vi "Control Panel Controller.vi"(8 "error in":errorcluster) -> ()   [LabVIEW 2020]
doc: "This VI executes continuously carrying out the current operation and responding to updates or new operations. It will often contain the timing or control code that is difficult to place directly in TeleOp. This VI generally opens all sensors and motors and isolates the rest of the robot code from knowing how the operations are carried out."
uses:
  Control Panel Operations.ctl
  Control Panel Setpoints.ctl
  <vilib>/Rock Robotics/Network Tables/NT Write Boolean.vi
  <vilib>/Rock Robotics/WPI/Framework/Completion Status.ctl
panel:
  in  "Interactive Values":T1
  out "Current\nCmd":string
  in  "Buttons":cluster{"Execute Cmd":bool, "Abort Cmd":bool}
  out "Command Timing":cluster{"Start Time (ms)":u32, "Iterations":i32}
  out "Status":T3
  # "Tip: It may be helpful to observe inputs and sensor values.\nYou may also want to display tuning or debugging controls."
  # "Interactive Command: You may fill in the settings for a command\nand schedule it with the Execute button. You can observe and abort\nany command while fine tuning the code for the controller."
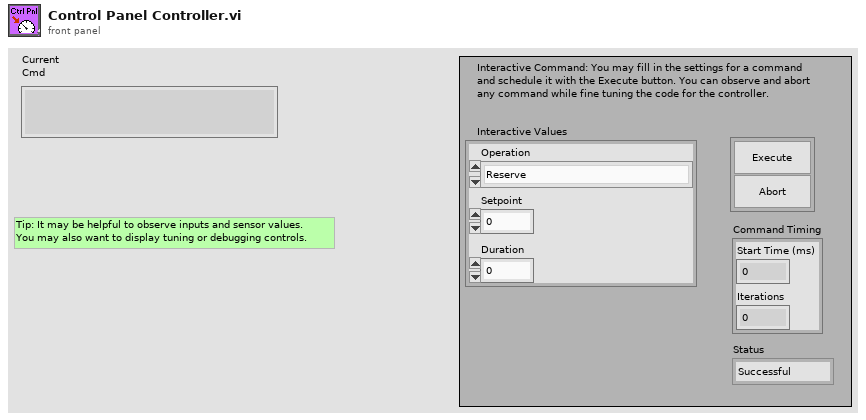
[diagram p1: front panel]
types:
  T1 = typedef "Control Panel Setpoints.ctl" = cluster{"Operation":T2, "Setpoint":dbl, "Duration":dbl}
  T2 = typedef "Control Panel Operations.ctl" = enum16{"Reserve", "Read Current", "Immediate", "Duration", "Stop"}
  T3 = typedef "Completion Status.ctl" = enum16{"Successful", "Aborted", "Incomplete"}
  T4 = typedef "Command Status Info.ctl" = cluster{"Name":string, "Status":T3, "notifier out":T5}
  T5 = typedef "Completion Notifier.ctl" = refnum<notifier>
  T6 = cluster{"Current Command":T1, "Command Timing":cluster{"Start Time (ms)":u32, "Iterations":i32}, "Command Arguments":cluster{"Command Info":T4, "Description":string, "Default Command":T1, "queue out":refnum<queue>, "Subsystem Name":string}}
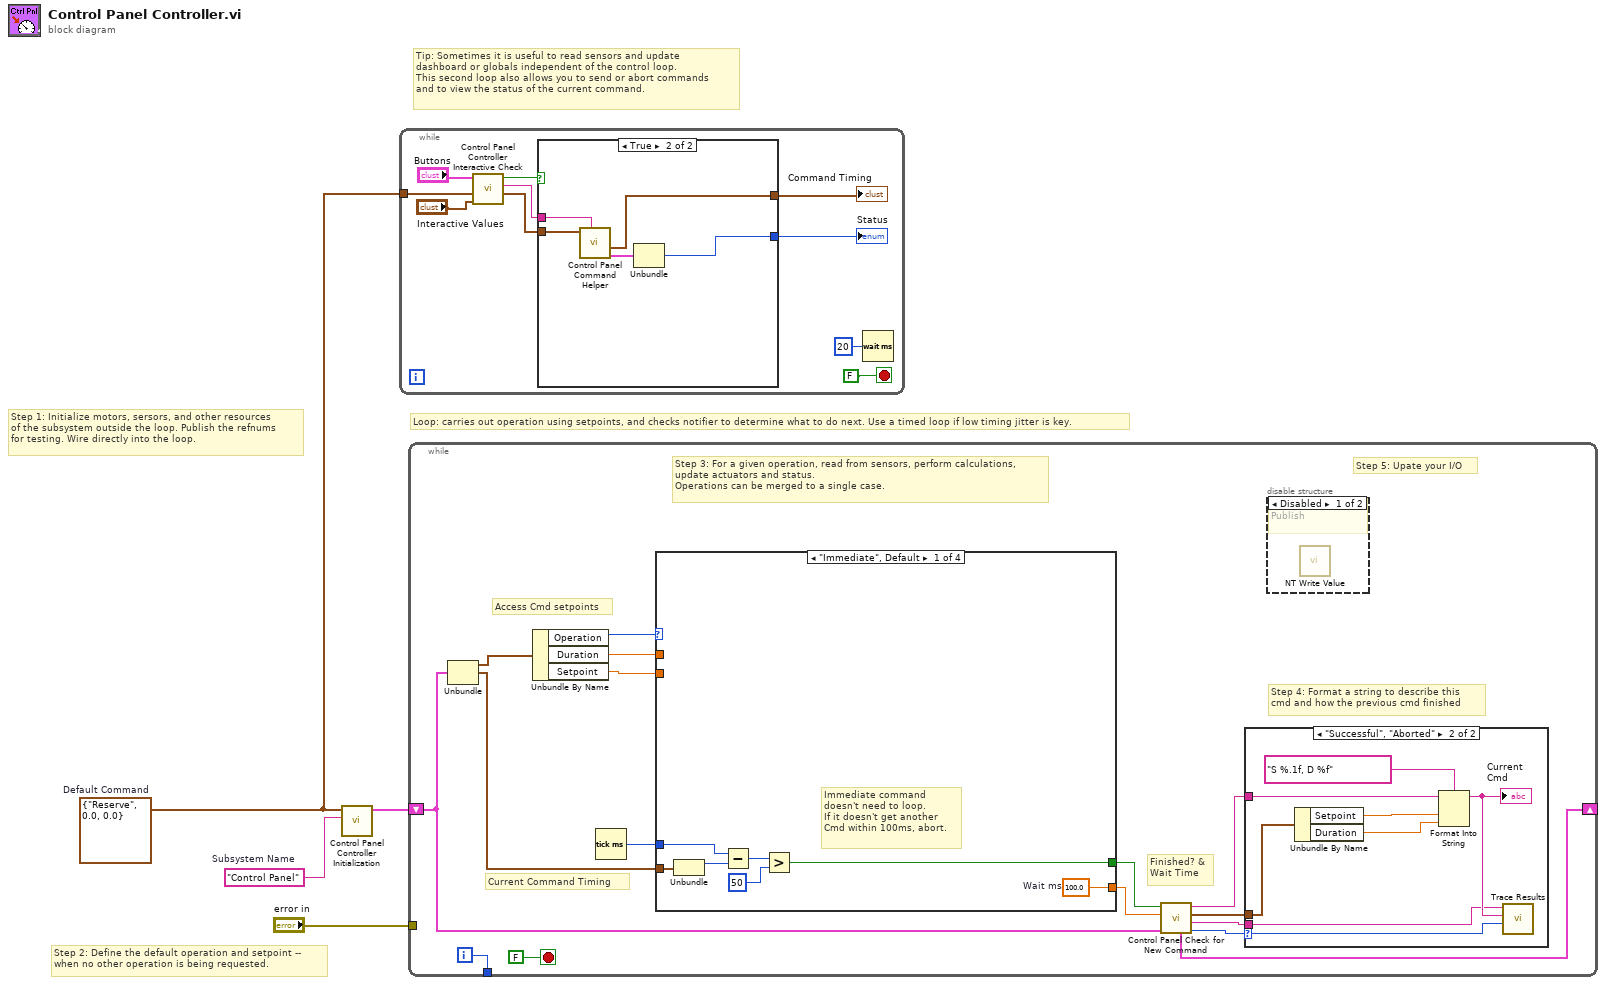
[diagram p0: block diagram]
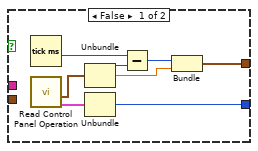
[diagram p2: hidden frame]
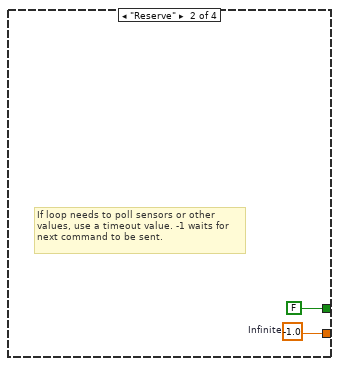
[diagram p5: hidden frame]
diagram:
  w1 = T1 {"Operation"=enum."Reserve", "Setpoint"=0.0, "Duration"=0.0}  # Default Command
  w2 = "Control Panel"  # Subsystem Name
  # "Tip: Sometimes it is useful to read sensors and update\ndashboard or globals independent of the control loop.\nThis second loop also allows you to send or abort commands\nand to view the status of the current command."
  # "Step 2: Define the default operation and setpoint --\nwhen no other operation is being requested."
  # "Step 1: Initialize motors, sersors, and other resources\nof the subsystem outside the loop. Publish the refnums\nfor testing. Wire directly into the loop."
  # "Loop: carries out operation using setpoints, and checks notifier to determine what to do next. Use a timed loop if low timing jitter is key."
  n1 = call "Control Panel Controller Initialization.vi"("Subsystem Name"=w2, "Default Command"=w1) -> ("Current Command"=w3:T6)  [unwired: 9 in]
  n2 = while {
    tunnel: w1 -> [w11]
    stop <- FALSE stop-if-true
    n3 = call "Control Panel Controller Interactive Check.vi"("Interactive Command in"="Interactive Values", "Default Command"=w11, "Buttons"="Buttons") -> ("Interactive Command out"=w8:T1, "Trace String"=w9:string, "Schedule"=w10:bool)  [unwired: 6 in]
    n4 = case shown="True" w10 {
      tunnel: [w22 w27] -> w7
      tunnel: w8 -> [_ w25]
      tunnel: [w18 w23] -> w6
      tunnel: w9 -> [_ w26]
      frame False {
        n5 = Tick Count (ms)() -> (millisecond timer value=w17:u32)
        n6 = call "Read Control Panel Operation.vi"() -> ("Command Info"=w15:T4, "SubSystem Data"=w16:T1)  [unwired: 9 in, 1 out]
        n7 = Unbundle(w16) -> ("Operation"=w21:T2, "Setpoint"=w19:dbl)  [unwired: 1 out]
        n8 = Unbundle(w15) -> ("Status"=w22:T3)  [unwired: 2 out]
        n9 = Subtract(x=w17, y=w21) -> (x-y=w20:u32)
        n10 = Bundle(w20, "Setpoint"=w19) -> (w18:cluster{u32, "Setpoint":dbl})  [unwired: 1 in]
      }
      frame True {
        n11 = call "Control Panel Command Helper.vi"("Description"=w26, "SubSystem Data"=w25) -> ("Command Info Out"=w24:T4, "Command Timing"=w23:cluster{"Start Time (ms)":u32, "Iterations":i32})  [unwired: 7 in, 1 out]
        n12 = Unbundle(w24) -> ("Status"=w27:T3)  [unwired: 2 out]
      }
    }
    "Status" <- w7
    "Command Timing" <- w6
    n13 = Wait (ms)(milliseconds to wait=u32 20) -> ()  [unwired: 1 out]
  }
  n14 = while {
    shift-right: [w35] -> _
    shift-left: w3 -> [w28]
    tunnel: [w42] -> _
    tunnel: "error in" -> [_]
    i -> [w42]
    stop <- FALSE stop-if-true
    # "Step 5: Upate your I/O"
    # "Step 4: Format a string to describe this\ncmd and how the previous cmd finished"
    # "Current Command Timing"
    # "Access Cmd setpoints"
    # "Finished? &\nWait Time"
    # "Step 3: For a given operation, read from sensors, perform calculations,\nupdate actuators and status.\nOperations can be merged to a single case."
    n15 = Unbundle(w28) -> ("Current Command"=w41:T1, "Command Timing"=w37:cluster{"Start Time (ms)":u32, "Iterations":i32})  [unwired: 1 out]
    n16 = Unbundle By Name(w41) -> ("Operation"=w40:T2, "Duration"=w39:dbl, "Setpoint"=w36:dbl)
    n17 = Tick Count (ms)() -> (millisecond timer value=w38:u32)
    n18 = case shown="\"Immediate\", Default" w40 {
      tunnel: [w58 w60 _ _] -> w33
      tunnel: [w52 FALSE ("ignore previous (F)") _ _] -> w34
      tunnel: w37 -> [w54 _ _ _]
      tunnel: w39 -> [_ _ _ _]
      tunnel: w38 -> [w53 _ _ _]
      tunnel: w36 -> [_ _ _ _]
      frame "Immediate", Default {
        w58 = 100.0  # Wait ms
        # "Immediate command\ndoesn't need to loop.\nIf it doesn't get another\nCmd within 100ms, abort."
        n19 = Unbundle(w54) -> ("Start Time (ms)"=w57:u32)  [unwired: 1 out]
        n20 = Subtract(x=w53, y=w57) -> (x-y=w56:u32)
        n21 = Greater?(x=w56, y=u8 50 ("Left Motor")) -> (0:w52:bool)
      }
      frame "Reserve" {
        w60 = -1.0  # Infinite
        # "If loop needs to poll sensors or other\nvalues, use a timeout value. -1 waits for\nnext command to be sent."
      }
      frame "Duration" {
      }
      frame "Stop" {
      }
    }
    n22 = call "Control Panel Check for New Command.vi"("Current Command"=w28, "Wait time (ms)"=w33, "Finished?"=w34) -> ("Completion"=w29:T3, "Subsystem Name"=w30:string, "Current Command"=w31:T1, "Initial Trace String"=w32:string, "NextCommand"=w35:T6)  [unwired: 4 in]
    n23 = case shown="\"Successful\", \"Aborted\"" w29 {
      selector: w29 -> [_ w51]
      tunnel: w32 -> [_ w47]
      tunnel: w31 -> [_ w48]
      tunnel: w30 -> [_ w44]
      frame "Incomplete", Default {
        # "Continuing current command"
      }
      frame "Successful", "Aborted" {
        # "Report and setup for next command"
        n24 = Unbundle By Name(w48) -> ("Setpoint"=w50:dbl, "Duration"=w45:dbl)
        n25 = Format Into String(format string="S %.1f, D %f", initial string=w47, w50, w45) -> (resulting string=w46:string)  [unwired: 1 in, 1 out]
        "Current\nCmd" <- w46
        n26 = call <vilib>:"Trace Results.vi"("Status of previous command"=w51, "Description"=w46, "Subsystem"=w44) -> ()  [unwired: 9 in]
      }
    }
    n27 = disable-structure shown="Disabled" {
      frame Disabled {
        # "Publish"
        n28 = call-poly <vilib>:"NT Write Value.vi"() -> ()  [unwired: 11 in, 1 out]
      }
      frame Enabled {
      }
    }
  }
